vi "Initiate.vi"(8 "error in (no error)":errorcluster, 11 "Agilent DSO1000 in":refnum<class "Agilent DSO1000.lvclass">) -> (0 "error out":errorcluster, 3 "Agilent DSO1000 out":refnum<class "Agilent DSO1000.lvclass">)   [LabVIEW 2020, in "Agilent DSO1000.lvclass"]
uses:
  Agilent DSO1000.lvclass
  C:/Sandbox/Git_Sandbox/WiSpry Test Framework source code (LV20)/WiSpry Test Framework/Instruments/Instrument.lvclass
  Instrument.lvclass/Instrument.ctl
  Instrument.lvclass
  <instrlib>/Agilent DSO1000 Series/Agilent DSO1000 Series.lvlib
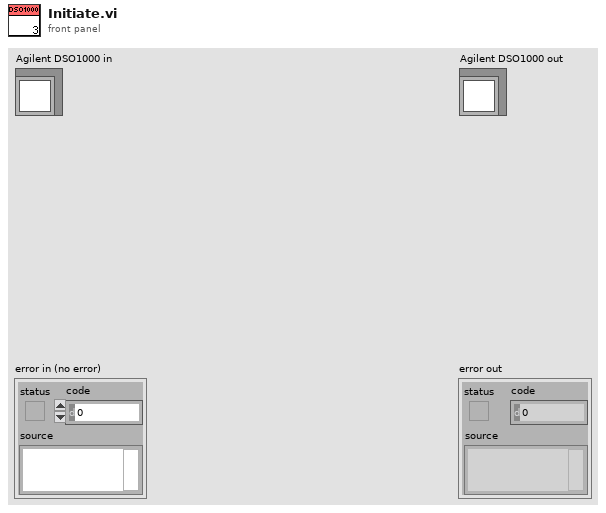
[diagram p1: front panel]
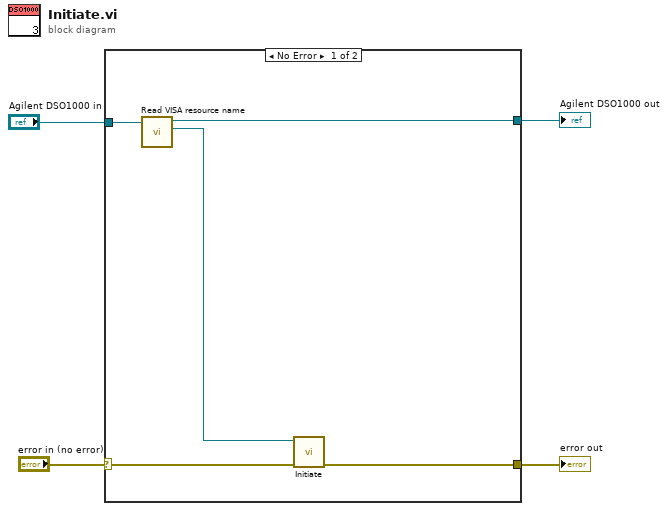
[diagram p0: block diagram]
diagram:
  n1 = case shown="No Error" "error in (no error)" {
    selector: "error in (no error)" -> [w8 w10]
    tunnel: [w5 w11] -> w3
    tunnel: "Agilent DSO1000 in" -> [w9 w11]
    tunnel: [w7 w10] -> w1
    frame No Error {
      n2 = call "Read VISA resource name.vi"("Instrument in"=w9) -> ("VISA resource name"=w6:refnum<visa-resource-name>, "Instrument out"=w5:refnum<class "Agilent DSO1000.lvclass">)  [unwired: 9 in]
      n3 = call <instrlib>:"Initiate.vi"("error in (no error)"=w8, "VISA resource name"=w6) -> ("error out"=w7:errorcluster)  [unwired: 8 in, 1 out]
    }
    frame Error {
    }
  }
  "error out" <- w1
  "Agilent DSO1000 out" <- w3
